vi "VerifWaveplate.vi"(8 "error in (no error)":errorcluster, 11 "Channel in":refnum<class "Channel.lvclass">) -> (0 "error out":errorcluster, 2 "OnePosition":bool, 3 "Channel out":refnum<class "Channel.lvclass">)   [LabVIEW 2018, in "Channel.lvclass"]
uses:
  Channel.lvclass
  Channel.lvclass/Channel.ctl
panel:
  out "log2(x)":dbl
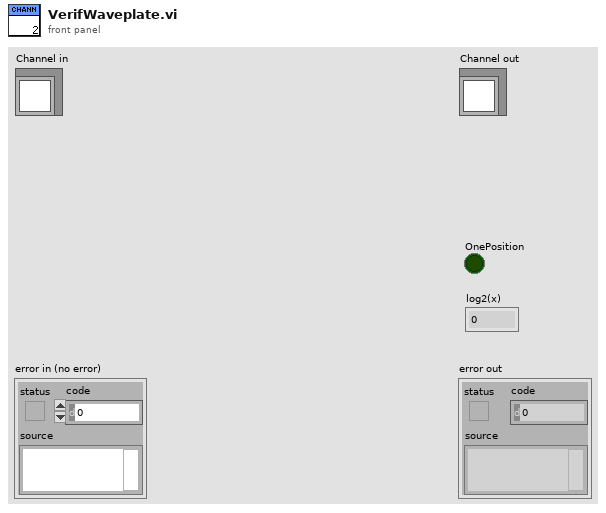
[diagram p1: front panel]
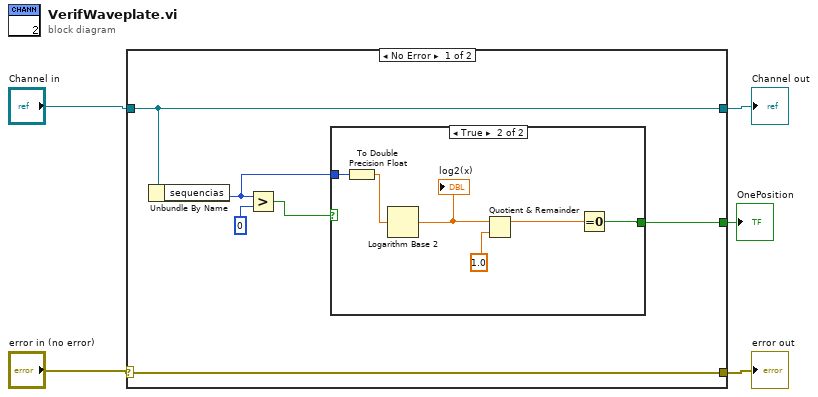
[diagram p0: block diagram]
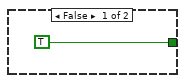
[diagram p2: hidden frame]
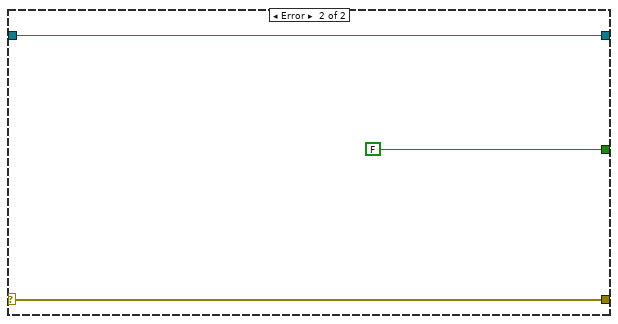
[diagram p3: hidden frame]
diagram:
  n1 = case shown="No Error" "error in (no error)" {
    selector: "error in (no error)" -> [w11 w21]
    tunnel: [w11 w21] -> w2
    tunnel: [w10 w20] -> w3
    tunnel: "Channel in" -> [w10 w20]
    tunnel: [w7 FALSE] -> w1
    frame No Error {
      n2 = Unbundle By Name(w10) -> ("sequencias"=w6:u32)
      n3 = Greater?(x=w6, y=u16 0) -> (0:w8:bool)
      n4 = case shown="True" w8 {
        tunnel: [TRUE w14] -> w7
        tunnel: w6 -> [_ w13]
        frame False {
        }
        frame True {
          n5 = To Double Precision Float(number=w13) -> (double precision float=w18:dbl)
          n6 = Logarithm Base 2(1:w18) -> (0:w15:dbl)
          "log2(x)" <- w15
          n7 = Quotient & Remainder(x=w15, y=1.0) -> (x-y*floor(x/y)=w17:dbl)  [unwired: 1 out]
          n8 = Equal To 0?(x=w17) -> (x = 0?=w14:bool)
        }
      }
    }
    frame Error {
    }
  }
  "error out" <- w2
  "Channel out" <- w3
  "OnePosition" <- w1
